vi "Generate_Arbitrary_Waveform_Sagar.vi"(4 "Channel (1|2)":u16, 5 "IP address":string, 6 "Frequency (1000 Hz)":i32, 7 "Channel (0: 1)":i32, 9 "Channel (1|2) 2":u16, 10 "Amplitude":dbl, 11 "Array":dbl[](array[numeric])) -> ()   [LabVIEW 2020]
uses:
  <instrlib>/Red_Pitaya/RedPitaya.lvlib
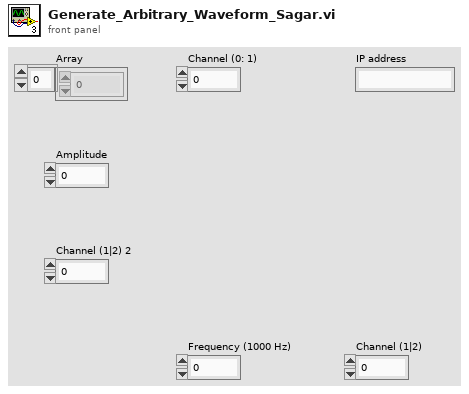
[diagram p1: front panel]
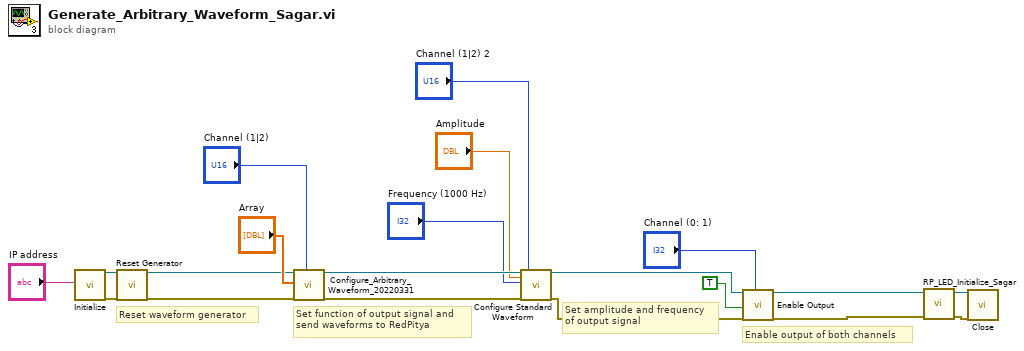
[diagram p0: block diagram]
diagram:
  # "Reset waveform generator"
  # "Enable output of both channels"
  # "Set amplitude and frequency\nof output signal"
  # "Set function of output signal and\nsend waveforms to RedPitya"
  n1 = call <instrlib>:"Initialize.vi"("IP address"="IP address") -> ("RedPitaya connection out"=w6:refnum<k5>, "error out"=w5:errorcluster)  [unwired: 17 in]
  n2 = call <instrlib>:"Reset Generator.vi"("RedPitaya connection in"=w6, "error in"=w5) -> ("RedPitaya connection out"=w16:refnum<k5>, "error out"=w17:errorcluster)  [unwired: 16 in]
  n3 = call "Configure_Arbitrary_Waveform_20220331.vi"("RedPitaya connection in"=w16, "Data"="Array", "error in"=w17, "Channel #"="Channel (1|2)") -> ("RedPitaya connection out"=w19:refnum<k5>, "error out"=w18:errorcluster)  [unwired: 14 in]
  n4 = call <instrlib>:"Configure Standard Waveform.vi"("RedPitaya connection in"=w19, "Amplitude (V)"="Amplitude", "Frequency"="Frequency (1000 Hz)", "error in"=w18, "Channel #"="Channel (1|2) 2") -> ("RedPitaya connection out"=w9:refnum<k5>, "error out"=w10:errorcluster)  [unwired: 13 in]
  n5 = call <instrlib>:"Enable Output.vi"("RedPitaya connection in"=w9, "Generation (T: Enable)"=TRUE, "error in"=w10, "Channel #"="Channel (0: 1)") -> ("RedPitaya connection out"=w4:refnum<k5>, "error out"=w1:errorcluster)  [unwired: 14 in]
  n6 = call "RP_LED_Initialize_Sagar.vi"("error in (no error)"=w1, "TCP Network Connection in"=w4) -> ("error out"=w2:errorcluster, "TCP Network Connection out"=w3:refnum<k5>)  [unwired: 8 in]
  n7 = call <instrlib>:"Close.vi"("RedPitaya connection in"=w3, "error in"=w2) -> ()  [unwired: 17 in, 1 out]
